vi "ex_SplitPacketDataRow.vi"(6 "get additional item":bool, 7 "file_params":T1={"include col headings?"=TRUE, "x_columns"=0, "col headings always?"=TRUE, "time preference"=0, "hide col headings"=FALSE} {"time preference" items=["Absolute", "Relative"]; "x_columns" items=["None", "One", "Multiple"]}, 8 "error in (no error)":errorcluster, 9 "nChannels":i32, 10 "delimiter":string="\t", 11 "row":string) -> (0 "error out":errorcluster, 1 "additional item":string, 2 "y strings":string[](array[string]), 3 "x strings":string[](array[string]))   [LabVIEW 2017]
uses:
  <vilib>/express/express input/ExFileReadBlock.llb/ex_ReadFileParams.ctl
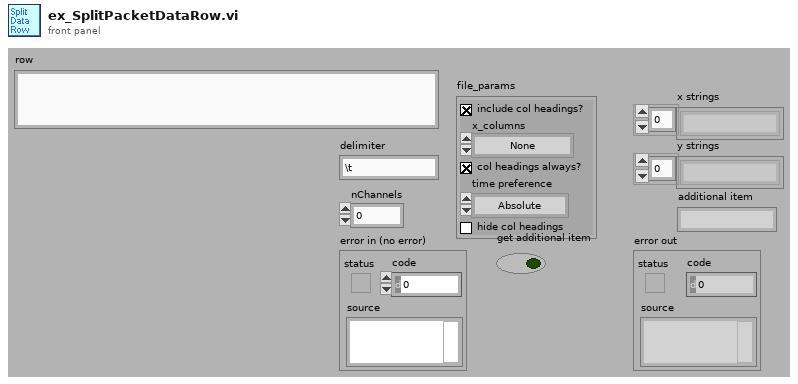
[diagram p1: front panel]
types:
  T1 = typedef "ex_ReadFileParams.ctl" = cluster{"include col headings?":bool, "x_columns":u16, "col headings always?":bool, "time preference":u16, "hide col headings":bool}
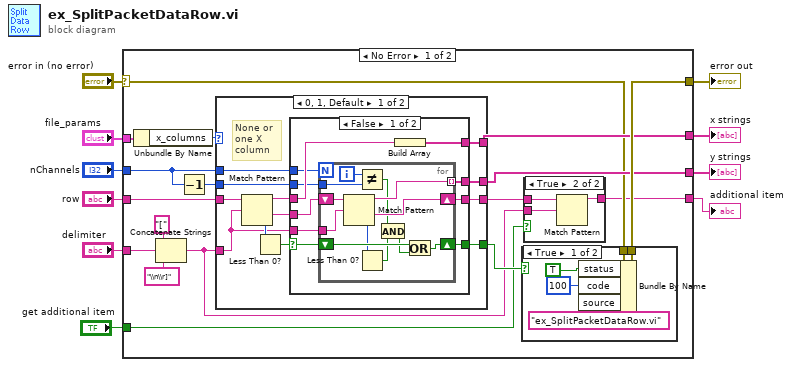
[diagram p0: block diagram]
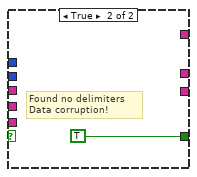
[diagram p4: hidden frame]
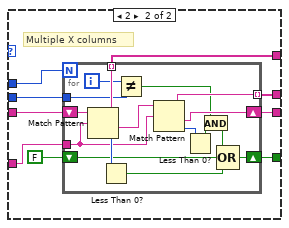
[diagram p5: hidden frame]
diagram:
  n1 = case shown="No Error" "error in (no error)" {
    selector: "error in (no error)" -> [w17 w97]
    tunnel: "file_params" -> [w27 _]
    tunnel: "delimiter" -> [w25 _]
    tunnel: "row" -> [w22 _]
    tunnel: [w21 w97] -> w7
    tunnel: [w19 _] -> w6
    tunnel: [w18 _] -> w5
    tunnel: "nChannels" -> [w16 _]
    tunnel: [w12 _] -> w2
    tunnel: "get additional item" -> [w11 _]
    frame No Error {
      n2 = Unbundle By Name(w27) -> ("x_columns"=w26:u16)
      n3 = Concatenate Strings("[", w25, "\\n\\r]") -> (w13:string)
      n4 = Decrement(x=w16) -> (x-1=w15:i32)
      n5 = case shown="0, 1, Default" w26 {
        tunnel: w22 -> [w48 w79]
        tunnel: w13 -> [w39 w78]
        tunnel: [w45 w74] -> w20
        tunnel: [w42 w75] -> w19
        tunnel: [w41 w76] -> w18
        tunnel: w16 -> [w40 w80]
        tunnel: w15 -> [w38 w73]
        tunnel: [w37 w72] -> w14
        frame 0, 1, Default {
          # "None or\none X\ncolumn"
          n6 = Match Pattern(string=w48, regular expression=w39) -> (before substring=w43:string, after substring=w44:string, offset past match=w47:i32)  [unwired: 2 out]
          n7 = Less Than 0?(x=w47) -> (x < 0?=w46:bool)
          n8 = case shown="False" w46 {
            selector: w46 -> [w55 _]
            tunnel: [w52 TRUE] -> w45
            tunnel: w44 -> [w54 _]
            tunnel: w43 -> [w58 _]
            tunnel: [w57 _] -> w42
            tunnel: [w53 _] -> w41
            tunnel: w40 -> [w56 _]
            tunnel: w39 -> [w51 _]
            tunnel: w38 -> [w50 _]
            tunnel: [w49 _] -> w37
            frame False {
              n9 = for {
                N: w56 -> [_]
                shift-right: [w66] -> w52
                shift-left: w55 -> [w67]
                shift-right: [w69] -> w49
                shift-left: w54 -> [w70]
                tunnel: [w68] -> w53 mode=indexing
                tunnel: w51 -> [w65]
                tunnel: w50 -> [w64]
                i -> [w63]
                n10 = Match Pattern(string=w70, regular expression=w65) -> (before substring=w68:string, after substring=w69:string, offset past match=w62:i32)  [unwired: 2 out]
                n11 = Not Equal?(x=w63, y=w64) -> (x != y?=w60:bool)
                n12 = Less Than 0?(x=w62) -> (x < 0?=w61:bool)
                n13 = And(x=w60, y=w61) -> (x .and. y?=w59:bool)
                n14 = Or(x=w67, y=w59) -> (x .or. y?=w66:bool)
              }
              n15 = Build Array(w58) -> (w57:string[])
            }
            frame True {
              # "Found no delimiters\nData corruption!"
            }
          }
        }
        frame 2 {
          # "Multiple X columns"
          n16 = for {
            N: w80 -> [_]
            shift-right: [w89] -> w74
            shift-left: FALSE -> [w88]
            shift-right: [w92] -> w72
            shift-left: w79 -> [w96]
            tunnel: [w86] -> w75 mode=indexing
            tunnel: w78 -> [w94]
            tunnel: [w91] -> w76 mode=indexing
            tunnel: w73 -> [w85]
            i -> [w84]
            n17 = Match Pattern(string=w96, regular expression=w94) -> (before substring=w86:string, after substring=w93:string, offset past match=w95:i32)  [unwired: 2 out]
            n18 = Less Than 0?(x=w95) -> (x < 0?=w87:bool)
            n19 = Not Equal?(x=w84, y=w85) -> (x != y?=w81:bool)
            n20 = Match Pattern(string=w93, regular expression=w94) -> (before substring=w91:string, after substring=w92:string, offset past match=w90:i32)  [unwired: 2 out]
            n21 = Less Than 0?(x=w90) -> (x < 0?=w82:bool)
            n22 = And(x=w81, y=w82) -> (x .and. y?=w83:bool)
            n23 = Compound Arithmetic op=OR(w83, w88, w87) -> (w89:bool)
          }
        }
      }
      n24 = case shown="True" w20 {
        tunnel: w17 -> [w35 w36]
        tunnel: [w32 w36] -> w21
        frame True {
          n25 = Bundle By Name(cluster=w35, "status"=TRUE, "code"=100, "source"="ex_SplitPacketDataRow.vi") -> (w32:errorcluster)
        }
        frame False {
        }
      }
      n26 = case shown="True" w11 {
        tunnel: w14 -> [_ w30]
        tunnel: w13 -> [_ w29]
        tunnel: [_ w28] -> w12
        frame False {
        }
        frame True {
          n27 = Match Pattern(string=w30, regular expression=w29) -> (before substring=w28:string)  [unwired: 4 out]
        }
      }
    }
    frame Error {
    }
  }
  "error out" <- w7
  "x strings" <- w6
  "y strings" <- w5
  "additional item" <- w2
